vi "calibration.vi"() -> ()   [LabVIEW 2017]
uses:
  <vilib>/FPGAPlugInAG/myRIO-1900/niLvFpga_Open_myRIO-1900.vi
  <vilib>/rvi/interface/common/dynamic/niFpgaDynamicAddResources.vi
  <vilib>/Utility/error.llb/Error Cluster From Error Code.vi
  <vilib>/rvi/errors/niLvFpgaAdjustHostInterfaceError.vi
  <vilib>/rvi/interface/nirviOpenFPGA/nirviOpenFPGA.xnode
  FPGA Bitfiles/PickleRio_FPGATarget_StepperFPGA2.0_025pYRGnFXk.lvbitx
  SubVI/Stepper FPGA 2.0.vi
  <vilib>/rvi/interface/nirviReadWriteControl/nirviReadWriteControl.xnode
  NiFpgaLv.dll
  <vilib>/rvi/interface/Simulation/niFpgaSimulationCallBeginRW.vi
panel:
  in  "stop":bool
  out "0?":bool
  in  "Pos":cluster{dbl, dbl, dbl, dbl, dbl, dbl, dbl, dbl}
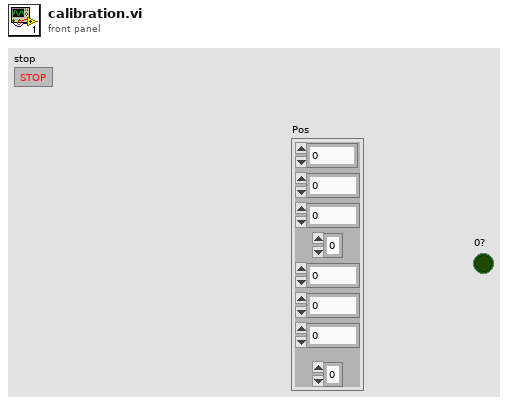
[diagram p1: front panel]
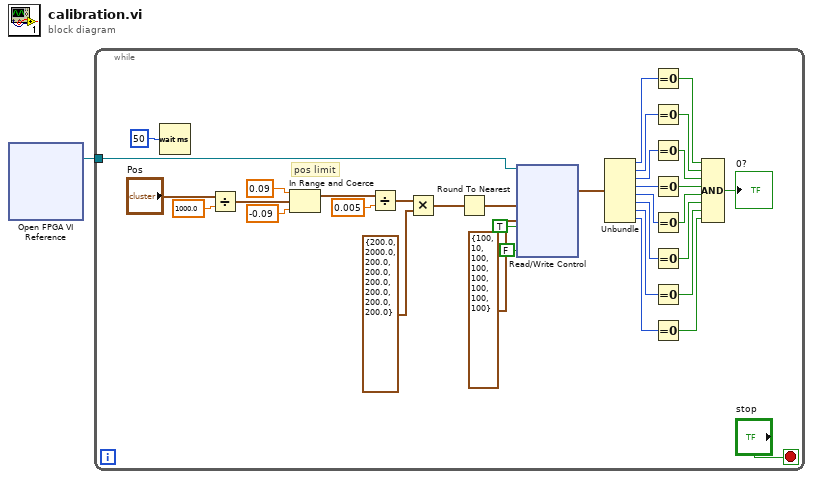
[diagram p0: block diagram]
diagram:
  n1 = xnode "Open FPGA VI Reference"() -> ("FPGA VI Reference Out"=w1:refnum<k20>)  [unwired: 2 in, 1 out]
  n2 = while {
    tunnel: w1 -> [w8]
    stop <- "stop" stop-if-true
    # "pos limit"
    n3 = Wait (ms)(milliseconds to wait=u32 50) -> ()  [unwired: 1 out]
    n4 = Divide(x="Pos", y=1000.0) -> (x/y=w10:cluster{dbl, dbl, dbl, dbl, dbl, dbl, dbl, dbl})
    n5 = In Range and Coerce(upper limit=0.09, x=w10, lower limit=-0.09) -> (coerced(x)=w31:cluster{dbl, dbl, dbl, dbl, dbl, dbl, dbl, dbl})  [unwired: 1 out]
    n6 = Divide(x=w31, y=0.005) -> (x/y=w32:cluster{dbl, dbl, dbl, dbl, dbl, dbl, dbl, dbl})
    n7 = Multiply(x=w32, y=cluster{dbl, dbl, dbl, dbl, dbl, dbl, dbl, dbl} {200.0, 2000.0, 200.0, 200.0, 200.0, 200.0, 200.0, 200.0}) -> (x*y=w36:cluster{dbl, dbl, dbl, dbl, dbl, dbl, dbl, dbl})
    n8 = Round To Nearest(number=w36) -> (nearest integer value=w6:cluster{dbl, dbl, dbl, dbl, dbl, dbl, dbl, dbl})
    n9 = xnode "Read/Write Control"("FPGA VI Reference In"=w8, "Steps"=w6, "Skipper"=cluster{i16, i16, i16, i16, i16, i16, i16, i16} {100, 10, 100, 100, 100, 100, 100, 100}, "Boolean"=TRUE, "Motors"=FALSE) -> ("Cluster"=w7:cluster{i16, i16, i16, i16, i16, i16, i16, i16})  [unwired: 1 in, 2 out]
    n10 = Unbundle(w7) -> (w30:i16, w29:i16, w28:i16, w27:i16, w26:i16, w25:i16, w24:i16, w23:i16)
    n11 = Equal To 0?(x=w30) -> (x = 0?=w22:bool)
    n12 = Equal To 0?(x=w29) -> (x = 0?=w21:bool)
    n13 = Equal To 0?(x=w28) -> (x = 0?=w20:bool)
    n14 = Equal To 0?(x=w27) -> (x = 0?=w19:bool)
    n15 = Equal To 0?(x=w26) -> (x = 0?=w18:bool)
    n16 = Equal To 0?(x=w25) -> (x = 0?=w17:bool)
    n17 = Equal To 0?(x=w24) -> (x = 0?=w16:bool)
    n18 = Equal To 0?(x=w23) -> (x = 0?=w15:bool)
    n19 = Compound Arithmetic op=AND(w22, w21, w20, w19, w18, w17, w16, w15) -> (→"0?":bool)
  }
